vi "get_calibration.vi"(8 "error in (no error)":errorcluster, 11 "Image.lvclass in":refnum<class "Image.lvclass">) -> (0 "error out":errorcluster, 1 "y":dbl, 2 "x":dbl, 3 "Image.lvclass out":refnum<class "Image.lvclass">, 4 "y unit":T1, 6 "x unit":T1)   [LabVIEW 2010, in "Image.lvclass"]
uses:
  Image.lvclass
  enumerations/unit.ctl
  Image.lvclass/Image.ctl
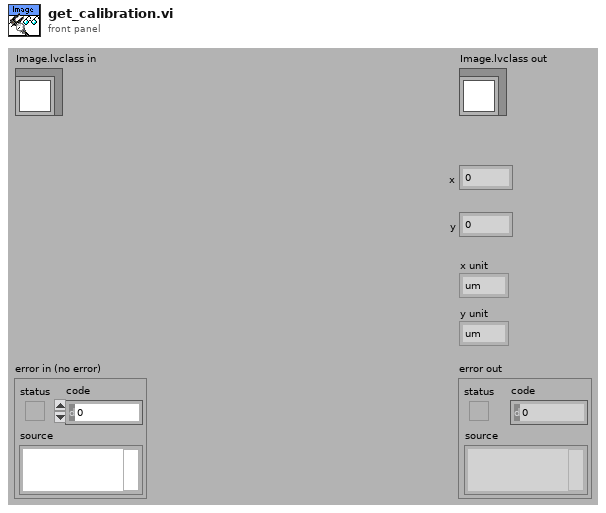
[diagram p1: front panel]
types:
  T1 = typedef "Image.lvclass/unit.ctl" = enum16{"um", "s"}
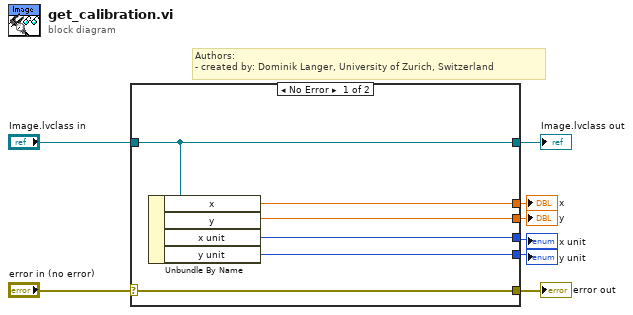
[diagram p0: block diagram]
diagram:
  # "Authors: \n- created by: Dominik Langer, University of Zurich, Switzerland"
  n1 = case shown="No Error" "error in (no error)" {
    selector: "error in (no error)" -> [w14 w15]
    tunnel: [w14 w15] -> w7
    tunnel: [w13 w16] -> w5
    tunnel: "Image.lvclass in" -> [w13 w16]
    tunnel: [w10 _] -> w3
    tunnel: [w9 _] -> w4
    tunnel: [w12 _] -> w2
    tunnel: [w11 _] -> w1
    frame No Error {
      n2 = Unbundle By Name(w13) -> ("x"=w10:dbl, "y"=w9:dbl, "x unit"=w12:T1, "y unit"=w11:T1)
    }
    frame Error {
    }
  }
  "error out" <- w7
  "Image.lvclass out" <- w5
  "y" <- w4
  "x" <- w3
  "y unit" <- w1
  "x unit" <- w2
